vi "Destroy.vi"(8 "error in (no error)":errorcluster, 11 "Result in":refnum<class "Task.lvclass">) -> (0 "error out":errorcluster)   [LabVIEW 2017, in "Futures.lvlib" / "Task.lvclass"]
uses:
  Task.lvclass
  Task.lvclass/Task.ctl
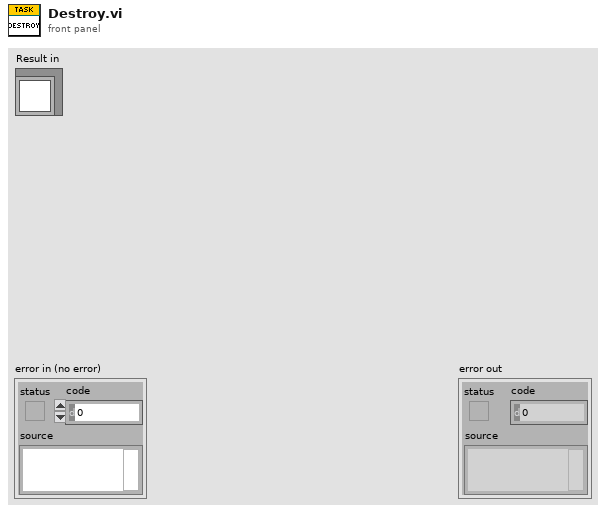
[diagram p1: front panel]
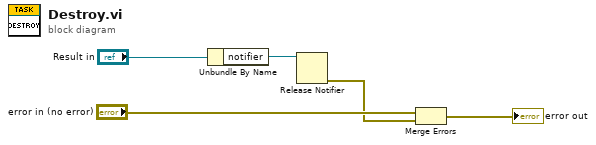
[diagram p0: block diagram]
diagram:
  n1 = Unbundle By Name("Result in") -> ("notifier"=w2:refnum<notifier>)
  n2 = Release Notifier(notifier=w2) -> (error out=w1:errorcluster)  [unwired: 2 in, 2 out]
  n3 = Merge Errors("error in (no error)", w1) -> (→"error out":errorcluster)
